vi "getTableAsDataRow.vi"(8 "error in (no error)":errorcluster, 11 "Transaction in":refnum<class "Transaction.lvclass">) -> (0 "error out":errorcluster, 3 "Table Row":string[](array[string]))   [LabVIEW 2018, in "Transaction.lvclass"]
uses:
  Transaction.lvclass
  Transaction.lvclass/Transaction.ctl
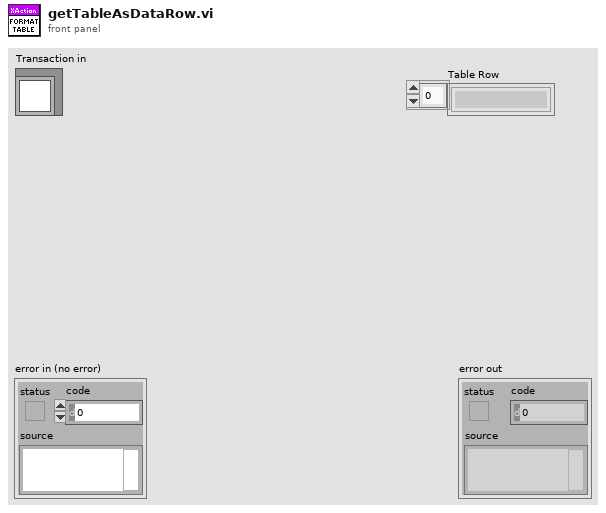
[diagram p1: front panel]
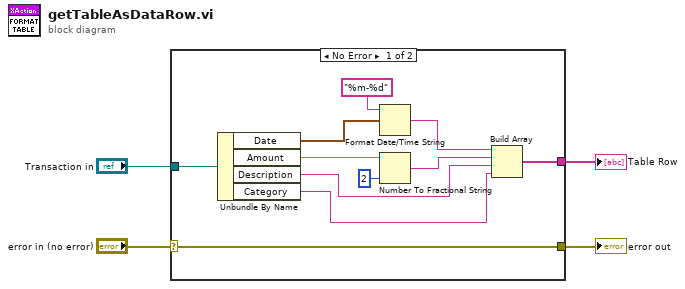
[diagram p0: block diagram]
diagram:
  n1 = case shown="No Error" "error in (no error)" {
    selector: "error in (no error)" -> [w15 w16]
    tunnel: [w15 w16] -> w3
    tunnel: "Transaction in" -> [w14 _]
    tunnel: [w9 _] -> w1
    frame No Error {
      n2 = Unbundle By Name(w14) -> ("Date"=w13:timestamp, "Amount"=w8:dbl, "Description"=w6:string, "Category"=w5:string)
      n3 = Format Date/Time String(time format string (%c)="%m-%d", seconds (now)=w13) -> (date/time string=w10:string)  [unwired: 1 in]
      n4 = Number To Fractional String(number=w8, precision (6)=i16 2) -> (F-format string=w7:string)  [unwired: 2 in]
      n5 = Build Array(w10, w7, w6, w5) -> (w9:string[])
    }
    frame Error {
    }
  }
  "error out" <- w3
  "Table Row" <- w1
